vi "OpenBase.vi"(5 "LogEnabled":bool, 7 "LogPath":path, 8 "error in (no error)":errorcluster, 9 "Instance":string, 10 "BaudRate":u32=125000, 11 "GenericCanAdapterClass in":refnum<class "GenericCanAdapterClass.lvclass">) -> (0 "error out":errorcluster, 3 "GenericCanAdapterClass out":refnum<class "GenericCanAdapterClass.lvclass">)   [LabVIEW 2011, in "GenericCanAdapterClass.lvclass"]
uses:
  GenericCanAdapterClass.lvclass
  GenericCanAdapterClass.lvclass/GenericCanAdapterClass.ctl
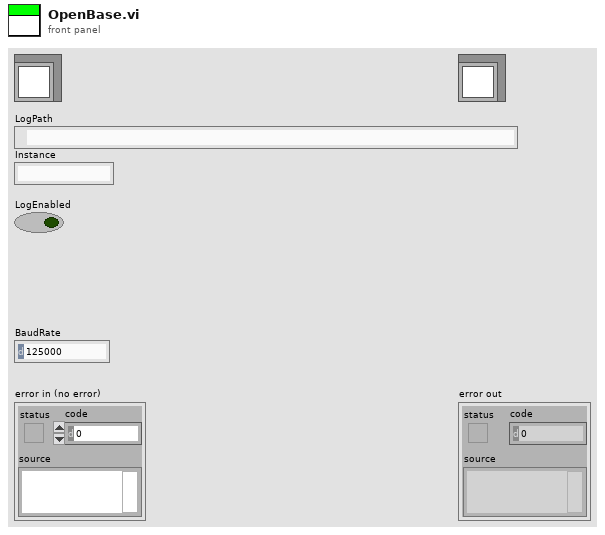
[diagram p1: front panel]
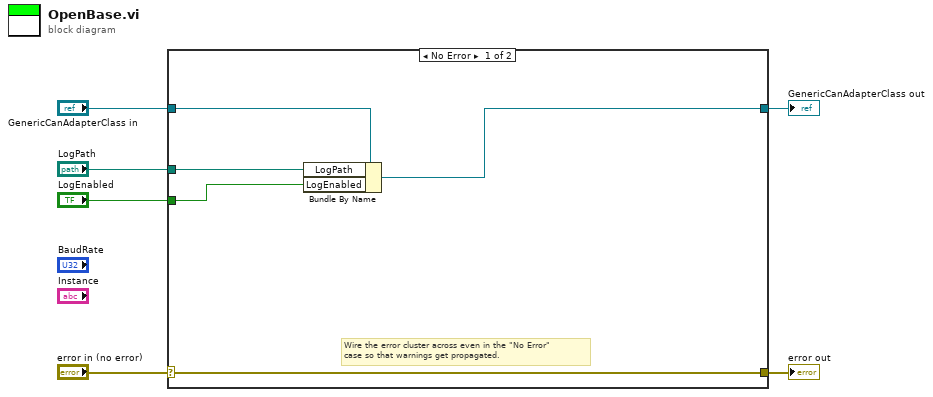
[diagram p0: block diagram]
diagram:
  n1 = case shown="No Error" "error in (no error)" {
    selector: "error in (no error)" -> [w11 w13]
    tunnel: [w11 w13] -> w5
    tunnel: [w9 w12] -> w3
    tunnel: "GenericCanAdapterClass in" -> [w10 w12]
    tunnel: "LogPath" -> [w8 _]
    tunnel: "LogEnabled" -> [w7 _]
    frame No Error {
      # "Wire the error cluster across even in the \"No Error\"\ncase so that warnings get propagated."
      n2 = Bundle By Name(cluster=w10, "LogPath"=w8, "LogEnabled"=w7) -> (w9:refnum<class "GenericCanAdapterClass.lvclass">)
    }
    frame Error {
    }
  }
  "error out" <- w5
  "GenericCanAdapterClass out" <- w3
